vi "Configure AFG Waveform Level.vi"(8 "error in (no error)":errorcluster, 9 "Low Level (-0.25 V)":dbl=-0.25, 10 "High Level (0.25 V)":dbl=0.25, 11 "VISA resource name":refnum<visa-resource-name>) -> (0 "error out":errorcluster, 3 "VISA resource name out":refnum<visa-resource-name>)   [LabVIEW 2017, in "Scope.lvlib" / "Tektronix DPO MSO 2000 4000 Series.lvlib"]
doc: "Configures the Arbitrary Function Generator high level and low level values of the output waveform.\n\n<B>Notes:</B>\n(1) This VI is available for MDO3000 Series only.\n\n(2) Requires the MDO3AFG option to be installed.\n\n(3) <B>Configure Output Impedance</B> VI must be used before this VI, so that saved setups are recalled with the proper load factor applied."
uses:
  Tektronix DPO MSO 2000 4000 Series.lvlib
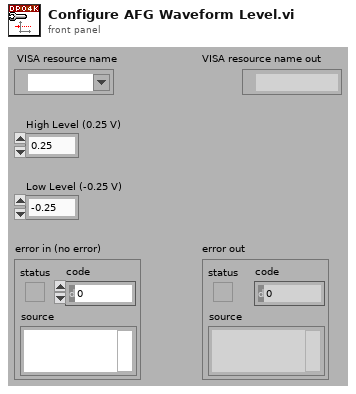
[diagram p1: front panel]
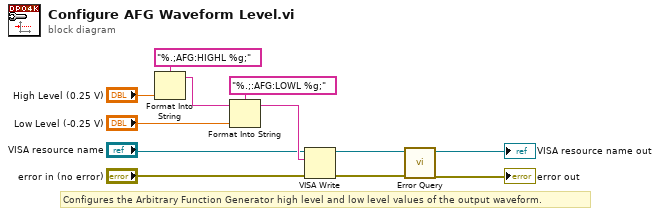
[diagram p0: block diagram]
diagram:
  # "Configures the Arbitrary Function Generator high level and low level values of the output waveform."
  n1 = Format Into String(format string="%.;AFG:HIGHL %g;", "High Level (0.25 V)") -> (resulting string=w10:string)  [unwired: 2 in, 1 out]
  n2 = Format Into String(format string="%.;:AFG:LOWL %g;", initial string=w10, "Low Level (-0.25 V)") -> (resulting string=w7:string)  [unwired: 1 in, 1 out]
  n3 = VISA Write(VISA resource name="VISA resource name", write buffer=w7, error in (no error)="error in (no error)") -> (VISA resource name out=w5:refnum<visa-resource-name>, error out=w4:errorcluster)  [unwired: 1 out]
  n4 = call "Error Query.vi"("error in (no error)"=w4, "VISA resource name"=w5) -> ("error out"=→"error out":errorcluster, "VISA resource name out"=→"VISA resource name out":refnum<visa-resource-name>)  [unwired: 6 in, 2 out]
